vi "overrideCount.vi"(8 "Error In":errorcluster, 11 "UI Elements Cluster":T1) -> (0 "Error Out":errorcluster)   [LabVIEW 2018]
uses:
  UI Module/src/controls/mainAppElementsCluster.ctl
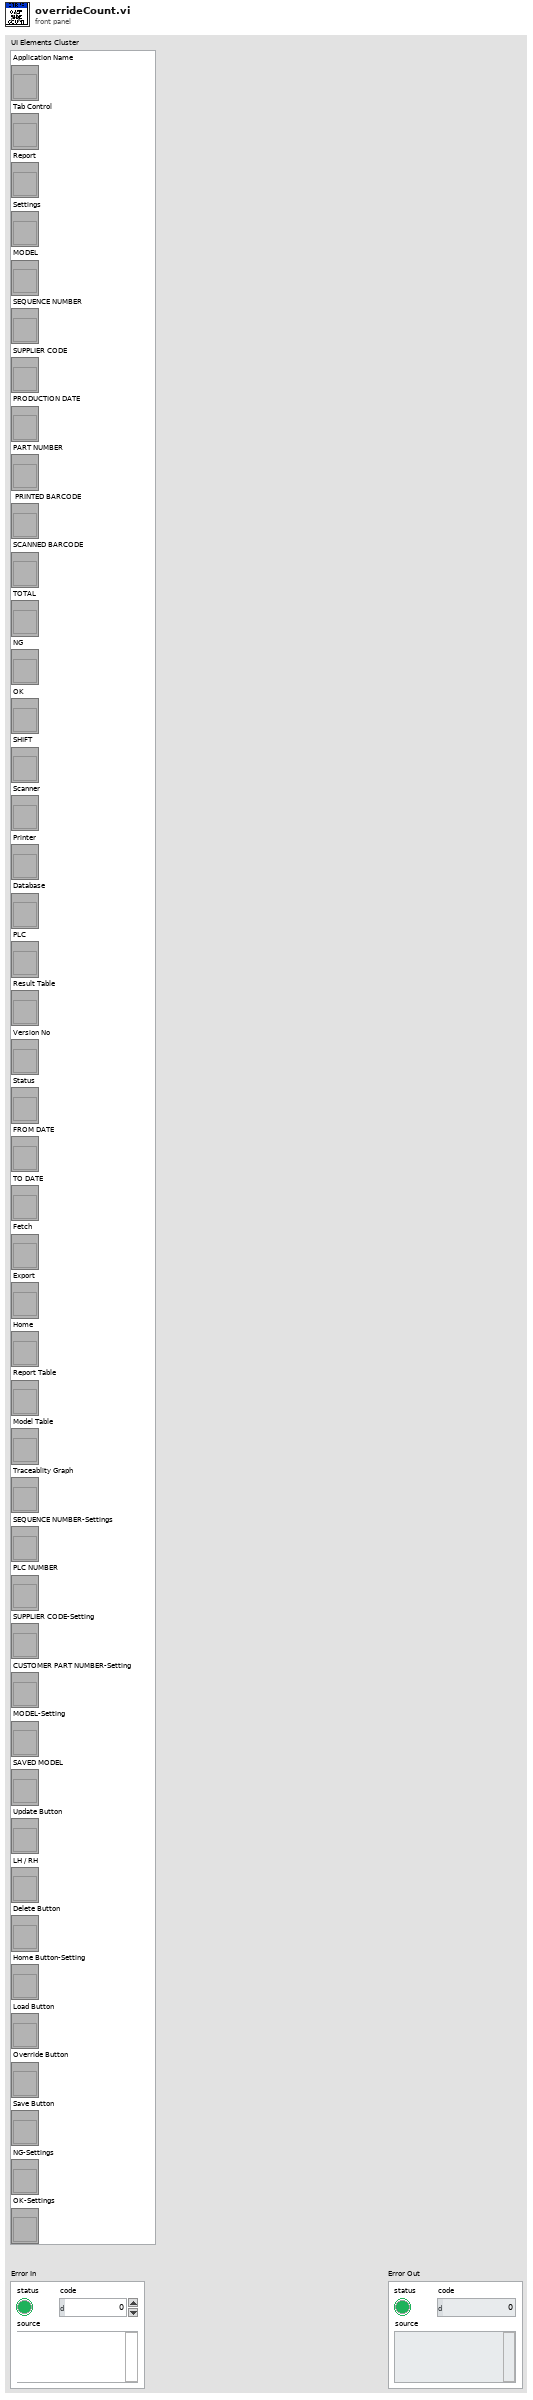
[diagram p1: front panel]
types:
  T1 = typedef "mainAppElementsCluster.ctl" = cluster{"Application Name":refnum<vi>, "Tab Control":refnum<vi>, "Status":refnum<vi>, "Version No":refnum<vi>, "Result Table":refnum<vi>, "PLC":refnum<vi>, "Database":refnum<vi>, "Printer":refnum<vi>, "Scanner":refnum<vi>, "SHIFT":refnum<vi>, "OK":refnum<vi>, "NG":refnum<vi>, "TOTAL":refnum<vi>, "SCANNED BARCODE":refnum<vi>, " PRINTED BARCODE":refnum<vi>, "PART NUMBER":refnum<vi>, "PRODUCTION DATE":refnum<vi>, "SUPPLIER CODE":refnum<vi>, "SEQUENCE NUMBER":refnum<vi>, "MODEL":refnum<vi>, "Settings":refnum<vi>, "Report":refnum<vi>, "Report Table":refnum<vi>, "Home":refnum<vi>, "Export":refnum<vi>, "Fetch":refnum<vi>, "TO DATE":refnum<vi>, "FROM DATE":refnum<vi>, "Model Table":refnum<vi>, "Traceablity Graph":refnum<vi>, "Override Button":refnum<vi>, "Load Button":refnum<vi>, "Home Button-Setting":refnum<vi>, "Delete Button":refnum<vi>, "Update Button":refnum<vi>, "Save Button":refnum<vi>, "SEQUENCE NUMBER-Settings":refnum<vi>, "PLC NUMBER":refnum<vi>, "LH / RH":refnum<vi>, "SUPPLIER CODE-Setting":refnum<vi>, "CUSTOMER PART NUMBER-Setting":refnum<vi>, "MODEL-Setting":refnum<vi>, "SAVED MODEL":refnum<vi>, "NG-Settings":refnum<vi>, "OK-Settings":refnum<vi>}
  T2 = cluster{"[0]":string, "[1]":string, "[2]":string, "[3]":string, "[4]":string, "[5]":string, "[6]":string, "[7]":string, "[8]":string}
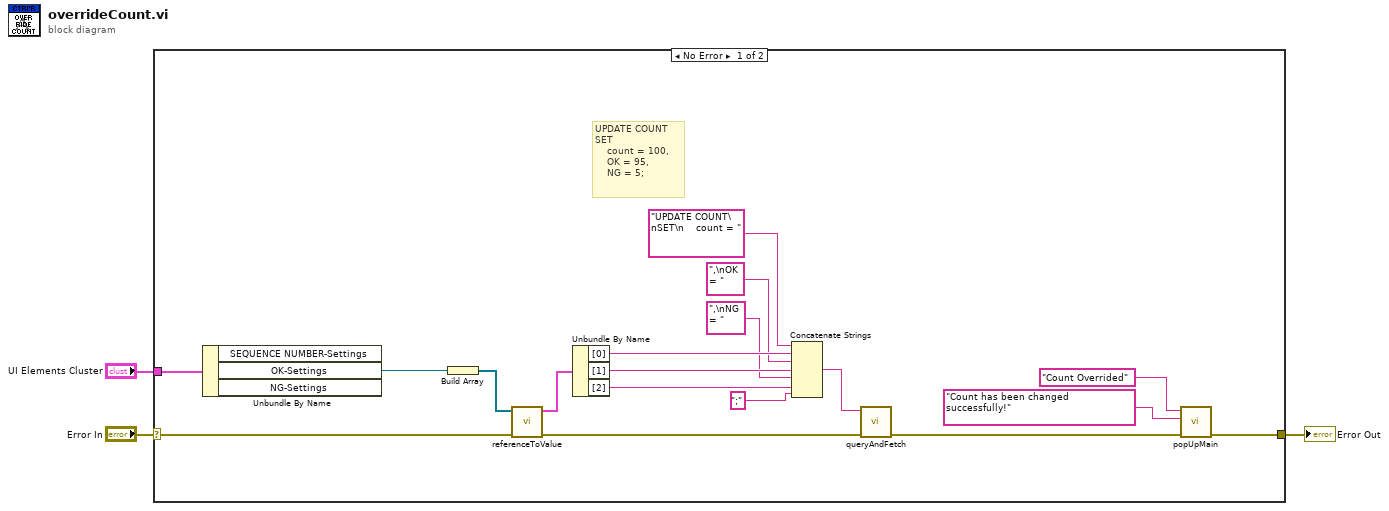
[diagram p0: block diagram]
diagram:
  n1 = case shown="No Error" "Error In" {
    selector: "Error In" -> [w19 w22]
    tunnel: [w16 w22] -> w2
    tunnel: "UI Elements Cluster" -> [w14 _]
    frame No Error {
      # "UPDATE COUNT\nSET\n    count = 100,\n    OK = 95,\n    NG = 5;"
      n2 = Unbundle By Name(w14) -> ("SEQUENCE NUMBER-Settings"=w21:refnum<vi>)  [unwired: 2 out]
      n3 = Build Array(w21) -> (w15:refnum<vi>[])
      n4 = call "referenceToValue.vi"("Error In"=w19, "Reference Array"=w15) -> ("Error Out"=w18:errorcluster, "Value Out Cluster"=w20:T2)  [unwired: 8 in]
      n5 = Unbundle By Name(w20) -> ("[0]"=w9:string, "[1]"=w7:string, "[2]"=w5:string)
      n6 = Concatenate Strings("UPDATE COUNT\nSET\n    count = ", w9, ",\nOK = ", w7, ",\nNG = ", w5, ";" ("string")) -> (w10:string)
      n7 = call "queryAndFetch.vi"("Error In"=w18, "Query"=w10) -> ("Error Out"=w17:errorcluster)  [unwired: 8 in, 1 out]
      n8 = call "popUpMain.vi"("Error In"=w17, "Message Description"="Count has been changed successfully!" ("Error Info"), "Message Titlt"="Count Overrided" ("Error Name")) -> ("Error Out"=w16:errorcluster)  [unwired: 7 in, 1 out]
    }
    frame Error {
    }
  }
  "Error Out" <- w2
